vi "test.vi"() -> ()   [LabVIEW 2016]
uses:
  APP/excelFile_class/fileType.ctl
  APP/excelFile_class/excelFile.lvclass
panel:
  in  "data":string[][][](array[string])
  in  "Boolean":bool
  in  "fileType":T1
  in  "Path":path
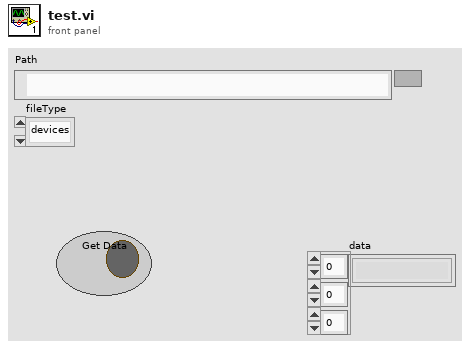
[diagram p1: front panel]
types:
  T1 = typedef "excelFile.lvclass/fileType.ctl" = enum16{"devices", "items", "partsTracking", "TSR"}
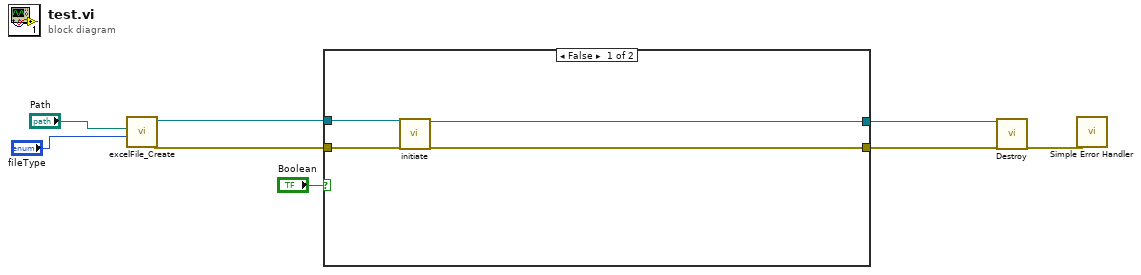
[diagram p0: block diagram]
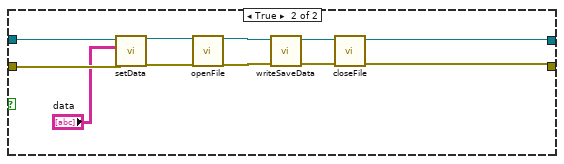
[diagram p2: hidden frame]
diagram:
  n1 = call "excelFile_Create.vi"("fileType"="fileType", "Path"="Path") -> ("error out"=w5:errorcluster, "reference out"=w6:refnum<class "excelFile.lvclass">)  [unwired: 8 in]
  n2 = case shown="False" "Boolean" {
    tunnel: w6 -> [w12 w23]
    tunnel: w5 -> [w11 w22]
    tunnel: [w10 w14] -> w4
    tunnel: [w9 w15] -> w3
    frame False {
      n3 = call-dynamic "initiate.vi"("reference in"=w12, "error in (no error)"=w11) -> ("reference out"=w10:refnum<class "excelFile.lvclass">, "error out"=w9:errorcluster)  [unwired: 16 in]
    }
    frame True {
      n4 = call "setData.vi"("error in (no error)"=w22, "data"="data", "reference in"=w23) -> ("error out"=w19:errorcluster, "reference out"=w21:refnum<class "excelFile.lvclass">)  [unwired: 7 in]
      n5 = call "openFile.vi"("reference in"=w21, "error in (no error)"=w19) -> ("reference out"=w20:refnum<class "excelFile.lvclass">, "error out"=w18:errorcluster)  [unwired: 16 in]
      n6 = call "writeSaveData.vi"("error in (no error)"=w18, "reference in"=w20) -> ("error out"=w16:errorcluster, "reference out"=w17:refnum<class "excelFile.lvclass">)  [unwired: 8 in]
      n7 = call "closeFile.vi"("error in (no error)"=w16, "reference in"=w17) -> ("error out"=w15:errorcluster, "reference out"=w14:refnum<class "excelFile.lvclass">)  [unwired: 8 in]
    }
  }
  n8 = call-dynamic "Destroy.vi"("reference in"=w4, "error in (no error)"=w3) -> ("error out"=w1:errorcluster)  [unwired: 16 in, 1 out]
  n9 = call <vilib>:"Simple Error Handler.vi"("error in (no error)"=w1) -> ()  [unwired: 4 in, 5 out]
